vi "loopTest.vi"() -> ()   [LabVIEW 2016]
uses:
  subVI/ZDataVIS_StateWire.ctl
  <vilib>/Utility/miscctls.llb/LVPointDoubleTypeDef.ctl
panel:
  out "X Linecut":cluster{"Vfast":dbl[], dbl[]}(graph) caption="XY Graph"
  out "Y Linecut":cluster{"Vfast":dbl[], dbl[]}(graph) caption="XY Graph"
  in  "State Wire IN":T1
  in  "show me the L O O P S":i32
  in  "2term Intensity":dbl[][](graph)
  # "cursor x"
  # "cursor y"
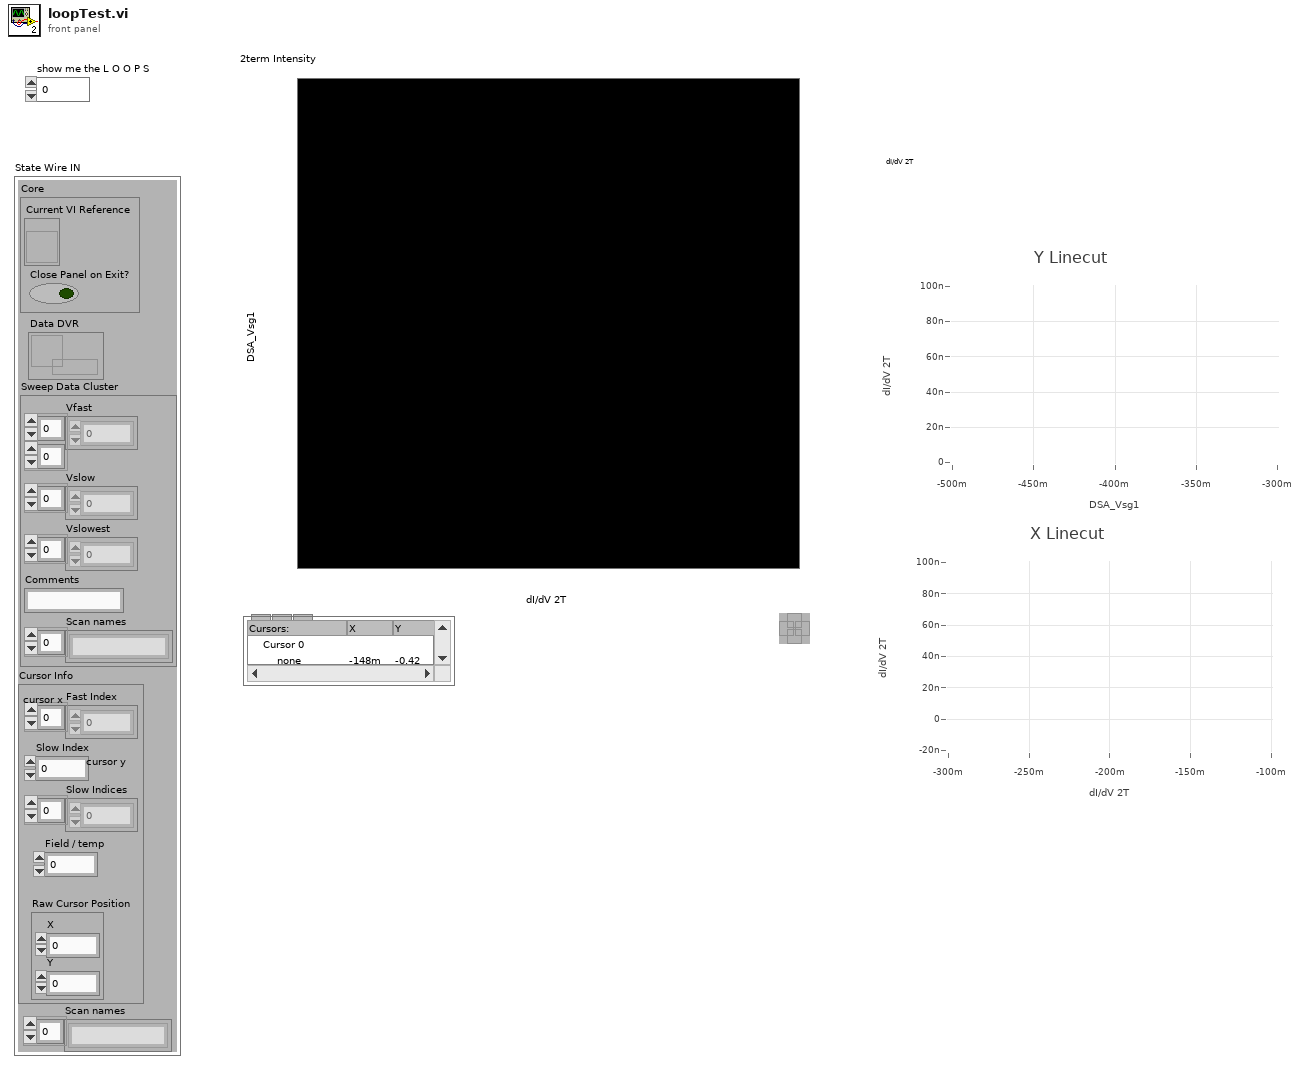
[diagram p1: front panel]
types:
  T1 = typedef "ZDataVIS_StateWire.ctl" = cluster{"Core":cluster{"Current VI Reference":refnum<vi>, "Close Panel on Exit?":bool}, "Sweep Data Cluster":cluster{"Vfast":dbl[][], "Vslow":dbl[], "Vslowest":dbl[], "Comments":string, "Scan names":string[]}, "Cursor Info":cluster{"Fast Index":dbl[], "Slow Index":dbl, "Slow Indices":dbl[], "Raw Cursor Position":T2, "Field / temp":i32}, "Scan names":string[], "Data DVR":refnum<data-value>}
  T2 = typedef "LVPointDoubleTypeDef.ctl" = cluster{"X":dbl, "Y":dbl}
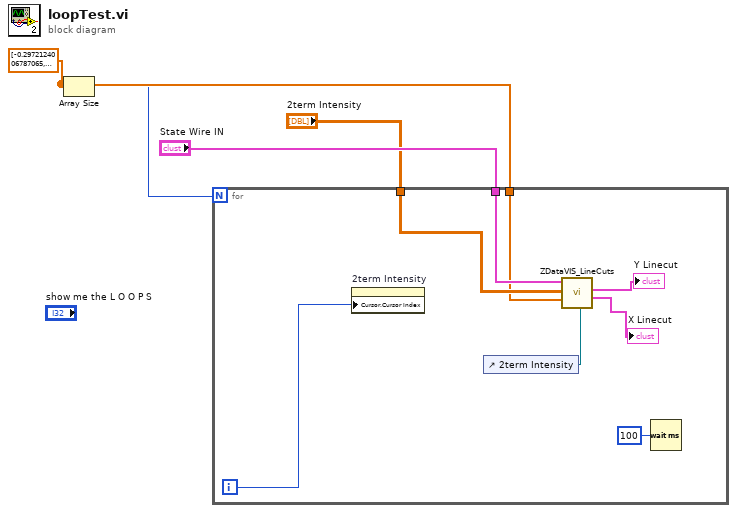
[diagram p0: block diagram]
diagram:
  w2 = dbl[] [-0.2972124006787065, -0.29522824542234977, -0.29324409016599295, -0.2912599349096362, -0.2892757796532794, -0.2872916243969226, -0.2853074691405658, -0.283323313884209, -0.2813391586278522, -0.27935500337149544, -0.2773708481151386, -0.27538669285878187, -0.27340253760242506, -0.2714183823460683, -0.2694342270897115, -0.2674500718333547, -0.2654659165769979, -0.2634817613206411, -0.2614976060642843, -0.25951345080792754, -0.2575292955515707, -0.25554514029521397, -0.25356098503885716, -0.25157682978250034, -0.24959267452614356, -0.24760851926978675, -0.24562436401342996, -0.24364020875707318, -0.2416560535007164, -0.2396718982443596, -0.2376877429880028, -0.235703587731646, -0.23371943247528923, -0.23173527721893242, -0.22975112196257566, -0.22776696670621885, -0.22578281144986206, -0.22379865619350528, -0.22181450093714847, -0.21983034568079168, -0.2178461904244349, -0.21586203516807811, -0.21387787991172133, -0.21189372465536452, -0.20990956939900773, -0.20792541414265095, -0.20594125888629414, -0.20395710362993738, -0.20197294837358057, -0.19998879311722378, -0.198004637860867, -0.1960204826045102, -0.19403632734815343, -0.19205217209179662, -0.19006801683543983, -0.18808386157908305, -0.18609970632272624, -0.18411555106636948, -0.18213139581001267, -0.18014724055365589, -0.1781630852972991, -0.1761789300409423, -0.1741947747845855, -0.17221061952822872, -0.17022646427187194, -0.16824230901551515, -0.16625815375915834, -0.16427399850280155, -0.16228984324644477, -0.16030568799008799, -0.15832153273373117, -0.1563373774773744, -0.1543532222210176, -0.15236906696466082, -0.15038491170830404, -0.14840075645194722, -0.14641660119559044, -0.14443244593923366, -0.14244829068287687, -0.14046413542652006, -0.13847998017016327, -0.1364958249138065, -0.1345116696574497, -0.13252751440109292, -0.1305433591447361, -0.12855920388837933, -0.12657504863202254, -0.12459089337566577, -0.12260673811930899, -0.12062258286295217, -0.11863842760659539, -0.1166542723502386, -0.11467011709388182, -0.11268596183752501, -0.11070180658116822, -0.10871765132481144, -0.10673349606845466, -0.10474934081209787, -0.10276518555574106, -0.10078103029938427] ("Decimated X values")
  n1 = Array Size(array=w2) -> (size(s)=w1:i32)
  n2 = for {
    N: w1 -> [_]
    tunnel: "State Wire IN" -> [w10]
    tunnel: "2term Intensity" -> [w9]
    tunnel: w2 -> [w8]
    i -> [w12]
    n3 = property on="2term Intensity" class="IntGraph (strict)"("Cursor.Cursor Index"=w12) -> ()  [unwired: 2 in, 2 out]
    n4 = control-ref of="2term Intensity"() -> (w5:refnum<vi>)
    n5 = call "ZDataVIS_LineCuts.vi"("Intensity Plot"=w5, "Decimated X values"=w8, "Arr of Y arrays (intensity info)"=w9, "State Wire IN"=w10) -> ("X line cut"=→"X Linecut":cluster{dbl[], dbl[]}, "Y line cut"=→"Y Linecut":cluster{"Vfast":dbl[], dbl[]})  [unwired: 4 in, 2 out]
    n6 = Wait (ms)(milliseconds to wait=u32 100) -> ()  [unwired: 1 out]
  }
